vi "init.vi"(4 "Current Cmd Data":variant, 5 "Subsystems":refnum<class>[](array[class]), 6 "Current Cmd":string, 7 "Command Determiner":refnum<vi>, 8 "error in (no error)":errorcluster, 9 "Valid Commands":refnum<class "Command.lvclass">[](array[class]), 10 "Name":string, 11 "Subsystem in":refnum<class "Subsystem.lvclass">) -> (0 "error out":errorcluster, 3 "Subsystem out":refnum<class "Subsystem.lvclass">)   [LabVIEW 2017, in "Subsystem.lvclass"]
uses:
  <userlib>/836-Library/Robot/Subsystem/Subsystem.lvclass
  <userlib>/836-Library/Robot/Command/Command.lvclass
  <userlib>/836-Library/Robot/Subsystem/Subsystem.lvclass/Subsystem.ctl
  <vilib>/ErrorRing/Error Ring.xnode
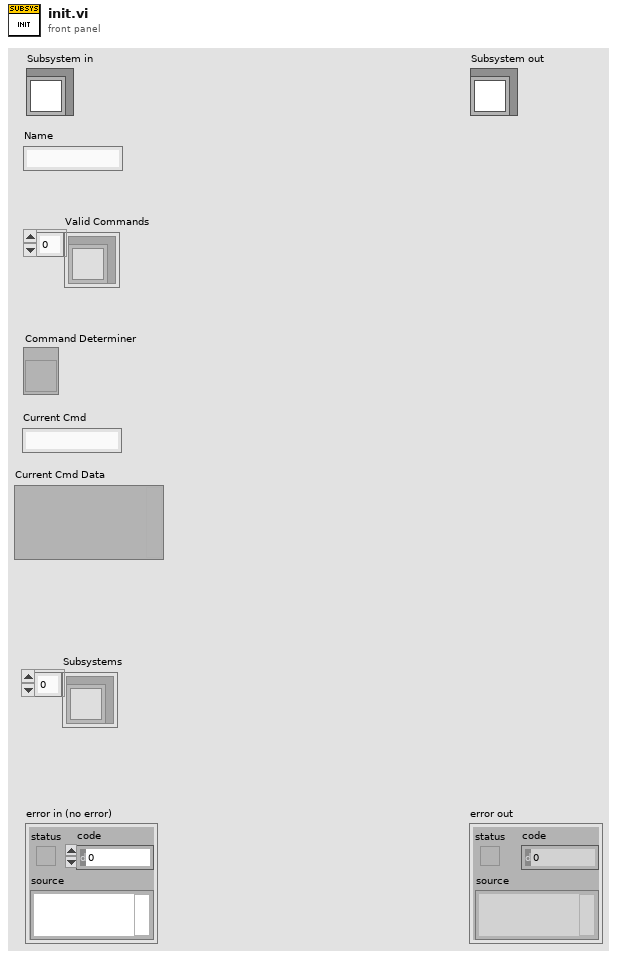
[diagram p1: front panel]
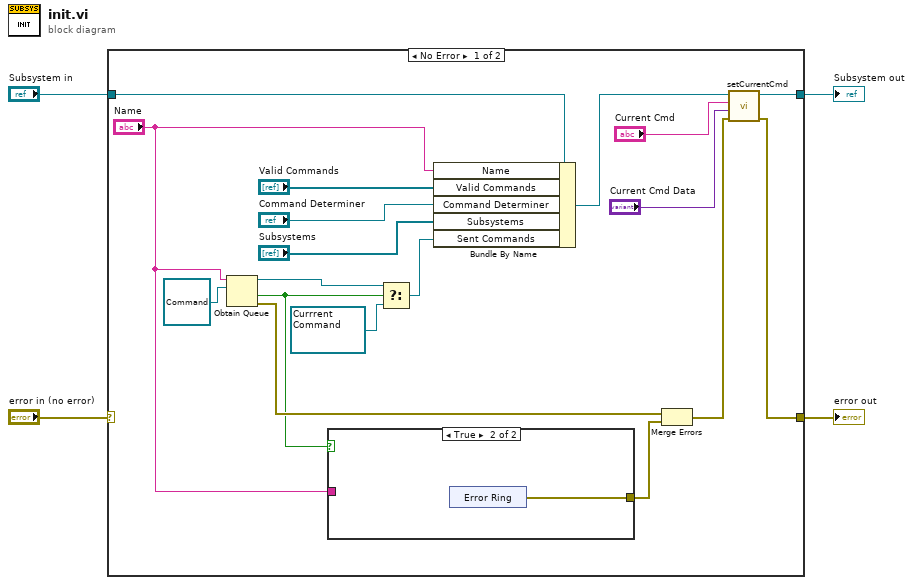
[diagram p0: block diagram]
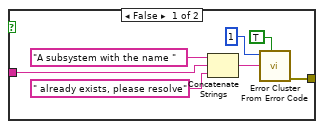
[diagram p2: hidden frame]
diagram:
  n1 = case shown="No Error" "error in (no error)" {
    selector: "error in (no error)" -> [_ w33]
    tunnel: [w5 w33] -> w3
    tunnel: [w8 w32] -> w1
    tunnel: "Subsystem in" -> [w22 w32]
    frame No Error {
      n2 = Obtain Queue(name (unnamed)="Name", element data type=refnum<class "Command.lvclass"> refnum ("Currrent Command")) -> (queue out=w18:refnum<queue>, created new?=w15:bool, error out=w16:errorcluster)  [unwired: 3 in]
      n3 = case shown="True" w15 {
        tunnel: [w28 w30] -> w14
        tunnel: "Name" -> [w25 _]
        frame False {
          n4 = Concatenate Strings("A subsystem with the name " ("string"), w25, " already exists, please resolve" ("string")) -> (w23:string)
          n5 = call <vilib>:"Error Cluster From Error Code.vi"("show call chain? (False)"=TRUE, "error message (\"\")"=w23, "error code (0)"=1) -> ("error out"=w28:errorcluster)  [unwired: 6 in]
        }
        frame True {
          n6 = xnode "Error Ring"() -> ("error out"=w30:errorcluster)
        }
      }
      n7 = Select(t=w18, s=w15, f=refnum<queue> refnum ("queue out")) -> (s? t:f=w11:refnum<queue>)
      n8 = Bundle By Name(cluster=w22, "Name"="Name", "Valid Commands"="Valid Commands", "Command Determiner"="Command Determiner", "Subsystems"="Subsystems", "Sent Commands"=w11) -> (w9:refnum<class "Subsystem.lvclass">)
      n9 = Merge Errors(w16, w14) -> (w10:errorcluster)
      n10 = call-dynamic "setCurrentCmd.vi"("error in (no error)"=w10, "Data"="Current Cmd Data", "Name"="Current Cmd", "Subsystem in"=w9) -> ("error out"=w5:errorcluster, "Subsystem out"=w8:refnum<class "Subsystem.lvclass">)  [unwired: 6 in]
    }
    frame Error {
    }
  }
  "error out" <- w3
  "Subsystem out" <- w1
